vi "Copy Auxiliary Stuff.vi"(8 "error in":errorcluster, 10 "Build Destination Folder Path":path, 11 "lvProject folder path":path) -> (0 "error out":errorcluster)   [LabVIEW 2020]
doc: "This VI copies some auxiliary files from project to build. E.g. it copies config.ini, but only when it is not in the build folder yet, so the old setup is preserved from previous EXE run."
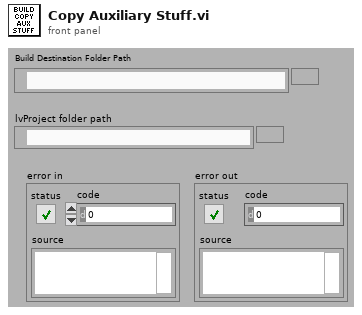
[diagram p1: front panel]
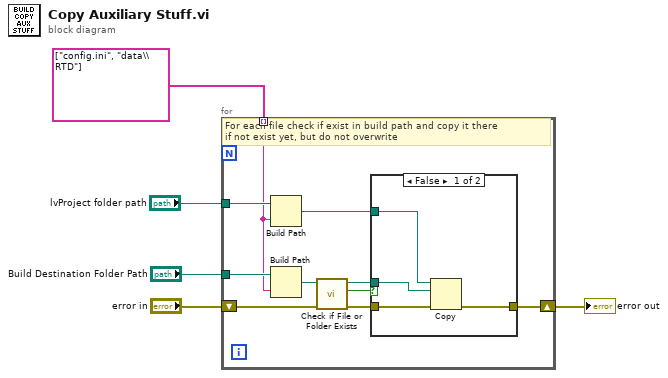
[diagram p0: block diagram]
diagram:
  n1 = for {
    tunnel: "Build Destination Folder Path" -> [w14]
    tunnel: string[] ["config.ini", "data\\RTD"] -> [w9] mode=indexing
    tunnel: "lvProject folder path" -> [w10]
    shift-right: [w6] -> w1
    shift-left: "error in" -> [w15]
    # "For each file check if exist in build path and copy it there\nif not exist yet, but do not overwrite"
    n2 = Build Path(base path=w10, name or relative path=w9) -> (appended path=w8:path)
    n3 = Build Path(base path=w14, name or relative path=w9) -> (appended path=w13:path)
    n4 = call <vilib>:"Check if File or Folder Exists.vi"("error in (no error)"=w15, "path"=w13) -> ("error out"=w11:errorcluster, "file or folder exists?"=w12:bool, "dup path"=w7:path)  [unwired: 7 in]
    n5 = case shown="False" w12 {
      tunnel: w11 -> [w19 w20]
      tunnel: w8 -> [w18 _]
      tunnel: w7 -> [w17 _]
      tunnel: [w16 w20] -> w6
      frame False {
        n6 = Copy(8:w19, 10:w17, 11:w18) -> (0:w16:errorcluster)  [unwired: 2 in, 2 out]
      }
      frame True {
      }
    }
  }
  "error out" <- w1
